vi "DOE Check Array Size.vi"(8 "Error In":errorcluster, 11 "Data List":dbl[](array[numeric])) -> (0 "Error Out":errorcluster, 3 "Output Array":dbl[](array[numeric]))   [LabVIEW 2016]
panel:
  out "Size Output":i32
  out "initialized array":dbl[](array[numeric])
  out "Size Input":i32
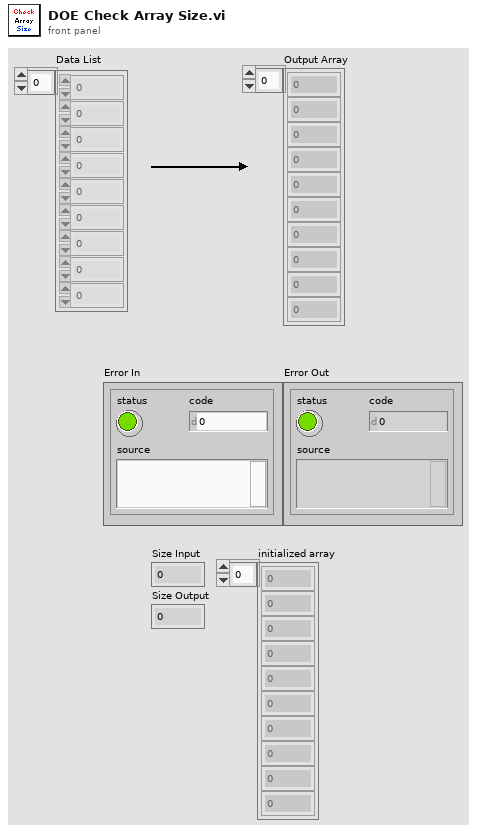
[diagram p1: front panel]
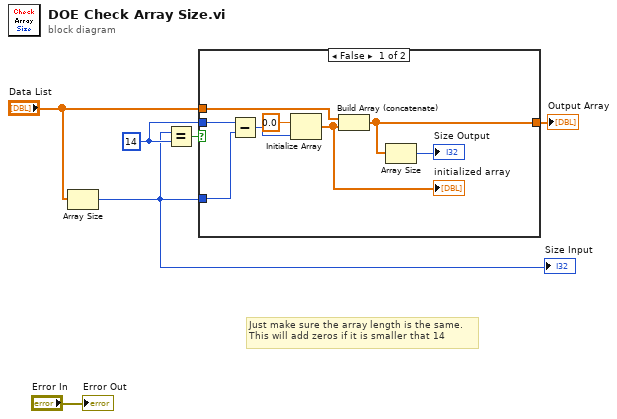
[diagram p0: block diagram]
diagram:
  w6 = 14 ("size(s) 2")
  # "Just make sure the array length is the same.\nThis will add zeros if it is smaller that 14"
  n1 = Array Size(array="Data List") -> (size(s)=w5:i32)
  "Size Input" <- w5
  n2 = Equal?(x=w5, y=w6) -> (x = y?=w2:bool)
  n3 = case shown="False" w2 {
    tunnel: w6 -> [w14 _]
    tunnel: w5 -> [w13 _]
    tunnel: "Data List" -> [w10 w15]
    tunnel: [w8 w15] -> w3
    frame False {
      n4 = Subtract(x=w14, y=w13) -> (x-y=w12:i32)
      n5 = Initialize Array(0.0, w12) -> (w9:dbl[])
      "initialized array" <- w9
      n6 = Build Array (concatenate)(w10, w9) -> (w8:dbl[])
      n7 = Array Size(array=w8) -> (size(s)=→"Size Output":i32)
    }
    frame True {
    }
  }
  "Output Array" <- w3
  "Error Out" <- "Error In"
